vi "Display Help for Selected Category.vi"(8 "error in (no error)":errorcluster, 11 "Configuration in":refnum<class "Configuration.lvclass">) -> (0 "error out":errorcluster, 3 "Configuration out":refnum<class "Configuration.lvclass">)   [LabVIEW 2020, in "Configuration.lvlib" / "Configuration.lvclass"]
uses:
  Configuration.lvclass
  Configuration.lvclass/Configuration.ctl
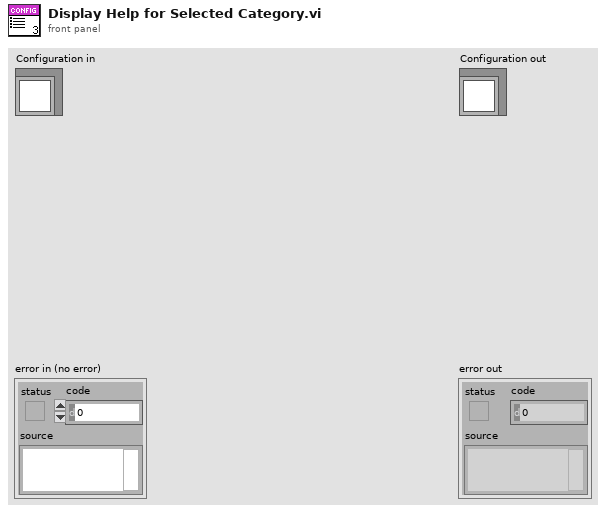
[diagram p1: front panel]
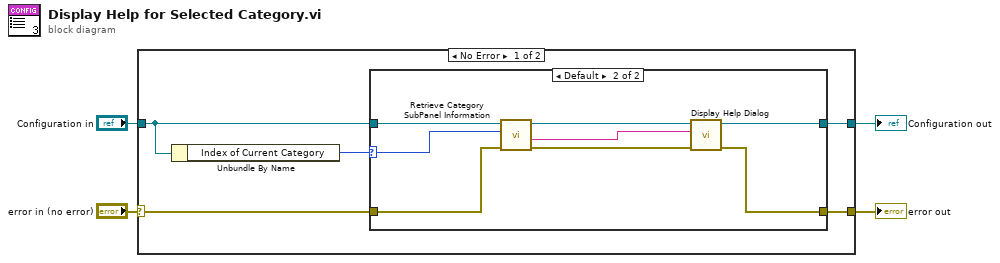
[diagram p0: block diagram]
diagram:
  n1 = case shown="No Error" "error in (no error)" {
    selector: "error in (no error)" -> [w7 w21]
    tunnel: [w6 w21] -> w3
    tunnel: [w8 w20] -> w1
    tunnel: "Configuration in" -> [w9 w20]
    frame No Error {
      n2 = Unbundle By Name(w9) -> ("Index of Current Category"=w5:i32)
      n3 = case shown="Default" w5 {
        selector: w5 -> [_ w12]
        tunnel: w9 -> [w11 w19]
        tunnel: [w11 w17] -> w8
        tunnel: w7 -> [w10 w14]
        tunnel: [w10 w13] -> w6
        frame -1 {
        }
        frame Default {
          n4 = call "Retrieve Category SubPanel Information.vi"("error in (no error)"=w14, "ListBox Selection"=w12, "Configuration in"=w19) -> ("error out"=w15:errorcluster, "Help Text"=w16:string, "Configuration Out"=w18:refnum<class "Configuration.lvclass">)  [unwired: 5 in, 1 out]
          n5 = call-dynamic "Display Help Dialog.vi"("error in (no error)"=w15, "Help Text"=w16, "Configuration in"=w18) -> ("error out"=w13:errorcluster, "Configuration out"=w17:refnum<class "Configuration.lvclass">)  [unwired: 7 in]
        }
      }
    }
    frame Error {
    }
  }
  "error out" <- w3
  "Configuration out" <- w1
